vi "Get Value.vi"(8 "error in (no error)":errorcluster, 11 "Descrambler in":refnum<class "Descrambler.lvclass">) -> (0 "error out":errorcluster, 2 "Value":i32, 3 "Descrambler out":refnum<class "Descrambler.lvclass">)   [LabVIEW 2020, in "Descrambler.lvclass"]
uses:
  Descrambler.lvclass
  Descrambler.lvclass/Descrambler.ctl
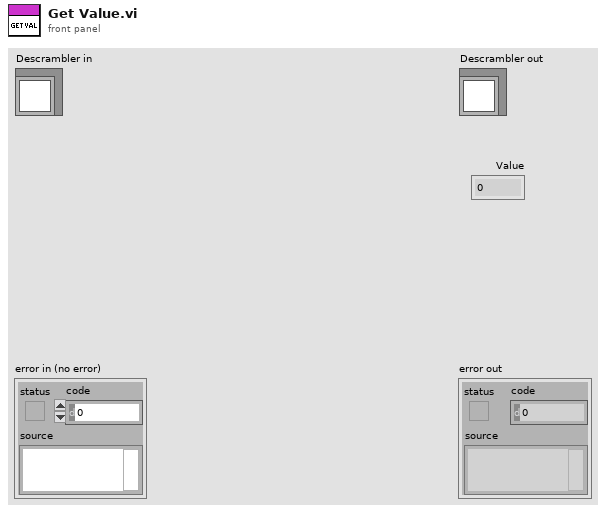
[diagram p1: front panel]
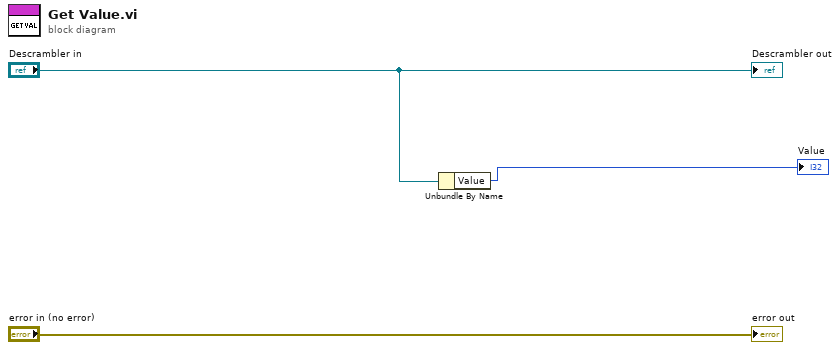
[diagram p0: block diagram]
diagram:
  n1 = Unbundle By Name("Descrambler in") -> ("Value"=→"Value":i32)
  "error out" <- "error in (no error)"
  "Descrambler out" <- "Descrambler in"
